vi "Create User Timestamps.vi"(0 "user timestamp data 0":fxp<+,58,58>, 1 "reset":bool, 5 "create user timestamp 0":bool, 7 "user timestamp data 1":fxp<+,58,58>, 9 "create user timestamp 1":bool) -> (4 "user timestamp fifo overflow":bool)   [LabVIEW 2020, in "GettingStarted_Acq_Tap_148X_FPGA.lvlib"]
uses:
  GettingStarted_Acq_Tap_148X_FPGA.lvlib
  <instrlib>/FlexRIO/CSI-2/v2/FPGA/Types/Timestamp ID.ctl
  <instrlib>/FlexRIO/CSI-2/v2/FPGA/subVIs/Convert User Timestamp to Raw Timestamp.vi
  <instrlib>/FlexRIO/CSI-2/v2/FPGA/subVIs/Pack Timestamps - x4.vi
  <instrlib>/_niInstr/Basic Elements/v1/FPGA/Private/Write U64 FIFO.vi
  <instrlib>/FlexRIO/CSI-2/v2/FPGA/NI CSI-2 API FPGA v2.lvlib
  <instrlib>/_niInstr/Basic Elements/v1/FPGA/niInstr Basic Elements v1 FPGA.lvlib
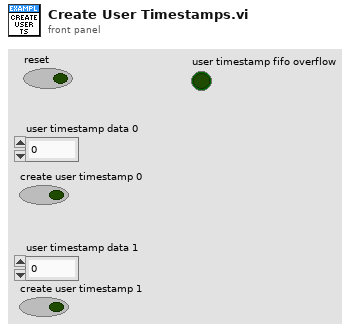
[diagram p1: front panel]
types:
  T1 = typedef "NI CSI-2 API FPGA v2.lvlib/Timestamp ID.ctl" = enum8{"SI0 LLP", "SI1 LLP", "SI2 LLP", "SI3 LLP", "SI4 LLP", "SI5 LLP", "SI6 LLP", "SI7 LLP", "SO0 LLP", "SO1 LLP", "SO2 LLP", "SO3 LLP", "SO4 LLP", "SO5 LLP", "SO6 LLP", "SO7 LLP", "Ser0 GPIO Bank", "Ser1 GPIO Bank", "Ser2 GPIO Bank", "Ser3 GPIO Bank", "Ser4 GPIO Bank", "Ser5 GPIO Bank", "Ser6 GPIO Bank", "Ser7 GPIO Bank", "Des0 GPIO Bank", "Des1 GPIO Bank", "Des2 GPIO Bank", "Des3 GPIO Bank", "Des4 GPIO Bank", "Des5 GPIO Bank", "Des6 GPIO Bank", "Des7 GPIO Bank", "User0", "User1", "User2", "User3", "User4", "User5", "User6", "User7", "User8", "User9", "User10", "User11", "User12", "User13", "User14", "User15", "User16", "User17", "User18", "User19", "User20", "User21", "User22", "User23", "User24", "User25", "User26", "User27", "User28", "User29", "User30", "User31"}
  T2 = typedef "NI CSI-2 API FPGA v2.lvlib/User Timestamp.ctl" = cluster{"valid":bool, "user data":fxp<+,58,58>, "id":T1}
  T3 = typedef "NI CSI-2 API FPGA v2.lvlib/Raw Timestamp.ctl" = cluster{"timestamp":u64, "valid":bool}
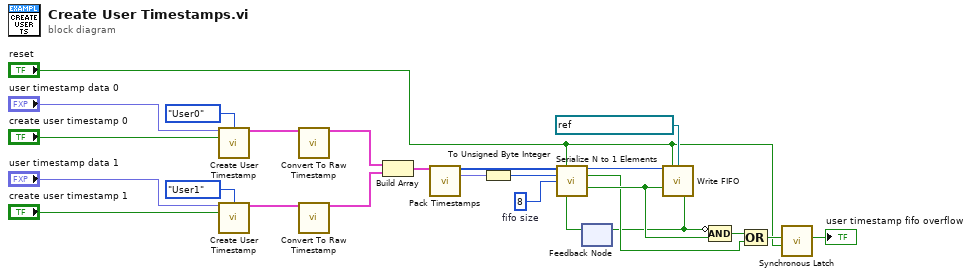
[diagram p0: block diagram]
diagram:
  w8 = u8 8  # fifo size
  n1 = call <instrlib>:"Create User Timestamp.vi"("user data"="user timestamp data 0", "timestamp id"=Timestamp_ID."User0", "create timestamp"="create user timestamp 0") -> ("user timestamp"=w22:T2)  [unwired: 12 in]
  n2 = call <instrlib>:"Create User Timestamp.vi"("user data"="user timestamp data 1", "timestamp id"=Timestamp_ID."User1", "create timestamp"="create user timestamp 1") -> ("user timestamp"=w24:T2)  [unwired: 12 in]
  n3 = call-poly <instrlib>:"Convert To Raw Timestamp.vi"("user timestamp"=w22) -> ("raw timestamp"=w23:T3)  [unwired: 14 in]
  n4 = call-poly <instrlib>:"Convert To Raw Timestamp.vi"("user timestamp"=w24) -> ("raw timestamp"=w25:T3)  [unwired: 14 in]
  n5 = Build Array(w23, w25) -> (w13:T3[])
  n6 = call-poly <instrlib>:"Pack Timestamps.vi"("timestamps in"=w13) -> ("valid timestamps"=w14:u64[], "num valid timestamps"=w15:fxp<+,3,3>)  [unwired: 13 in]
  n7 = To Unsigned Byte Integer(number=w15) -> (unsigned 8bit integer=w12:u8)
  n8 = feedback #1() -> (w9:bool)  [unwired: 1 in]
  n9 = call <instrlib>:"Serialize N to 1 Elements.vi"("elements in"=w14, "reset"="reset", "num elements in"=w12, "fifo size"=w8, "ready for output"=w9) -> ("element out"=w10:u64, "overflow"=w20:bool, "output valid"=w21:bool)  [unwired: 7 in, 1 out]
  n10 = call-poly <instrlib>:"Write FIFO.vi"("input data"=w10, "reset"="reset", "fifo"=refnum<k21> "User Timestamps" ("FIFO In"), "input valid"=w21) -> ("ready for input"=w19:bool)  [unwired: 11 in]
  n11 = feedback-in #1(w19) -> ()
  n12 = Compound Arithmetic op=AND(invert w19, w21) -> (w17:bool)
  n13 = Compound Arithmetic op=OR(w17, w20) -> (w16:bool)
  n14 = call <instrlib>:"Synchronous Latch.vi"("clear"="reset", "set"=w16) -> ("out"=→"user timestamp fifo overflow":bool)  [unwired: 9 in]
